vi "Pockels modulation task-Generate data.vi"(8 "error in (no error)":errorcluster, 11 "Setup/Logging queue element":T1={"Imaging Protocol"=enum."Live Imaging", "Number of Trials"=0, "Frame Size"=512, "# Averaged frames"=0, "Dwell time (us)"=0.0, "Index of Z-plane"=0, "Timelapse?"=FALSE, "Logging process is active"=FALSE, "Speed logging enabled"=FALSE, "tdms file ref"=refnum, "path"=path "", "Trial Number"=0, "Expected # points acquired"=FALSE, "Manually stopped"=FALSE, "Last trial"=FALSE, "Ch0 data"=[], "Ch1 data"=[], "Ref Data"=[], "Ref Frame Time"=[], "Image Time"=[], "Continuous Time"=[], "Ref X Length"=0, "Ref Y Length"=0, "# Ref Averaged frames"=0, "Ref Dwell time (us)"=0.0, "Points acquired"={"Ch0 last trial"=0, "Ch1 last trial"=0, "All trials"=0}, "HW Timings File"=refnum} {"Ref Dwell time (us)" format="%#.6g"; "Frame Size" items=["100X100"=100, "128X128"=128, "200X200"=200, "256X256"=256, "512X512"=512, "1024x1024"=1024, "2048x2048"=2048]; "Dwell time (us)" format="%#.6g"}) -> (0 "error":errorcluster, 1 "Data length (points)":i32, 2 "Pockels modulation data":dbl[](graph), 4 "Sampling period (us)":dbl format="%#_6f", 6 "Length of sequence (ms)":dbl format="%#_6f")   [LabVIEW 2020]
uses:
  Typedefs/Logging queue element.ctl
  Typedefs/Imaging Protocols enum.ctl
  Typedefs/Frame Size.ctl
  Typedefs/Acquired points count.ctl
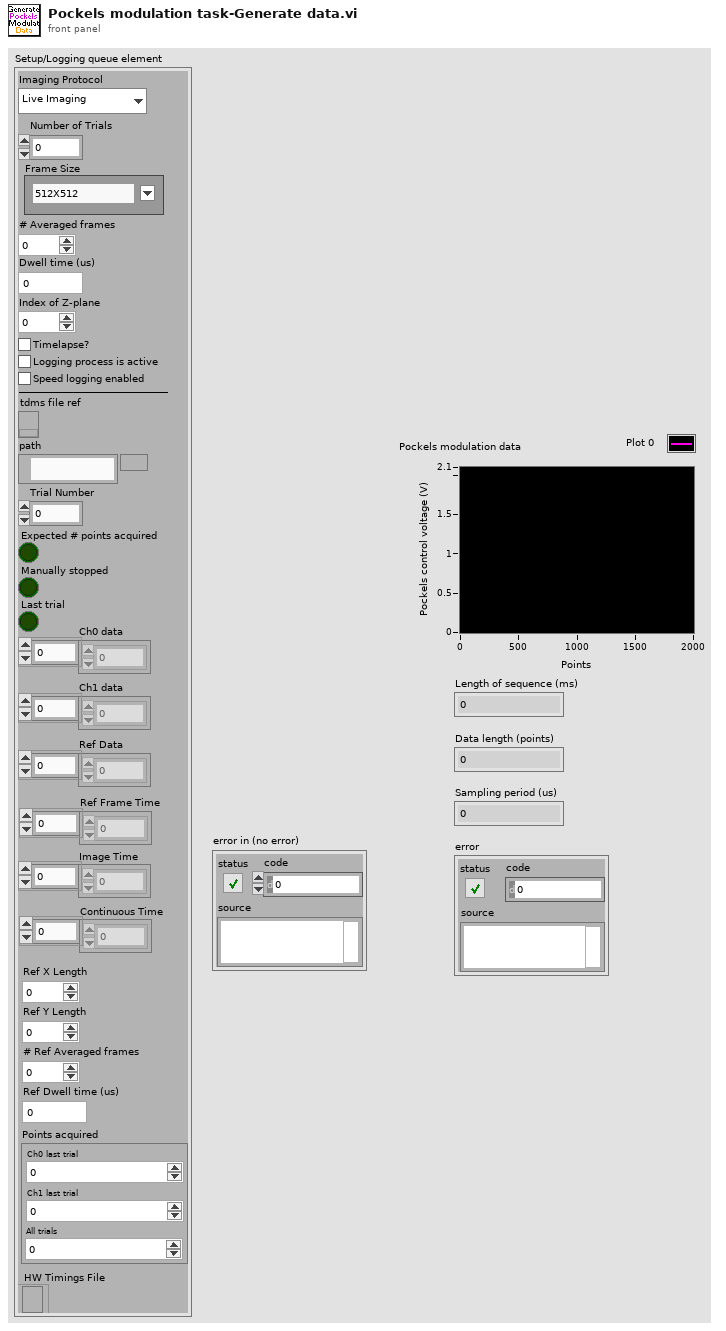
[diagram p1: front panel]
types:
  T1 = typedef "Logging queue element.ctl" = cluster{"Imaging Protocol":T2, "Number of Trials":u16, "Frame Size":T3, "# Averaged frames":u16, "Dwell time (us)":dbl, "Index of Z-plane":i32, "Timelapse?":bool, "Logging process is active":bool, "Speed logging enabled":bool, "tdms file ref":refnum<k34>, "path":path, "Trial Number":i32, "Expected # points acquired":bool, "Manually stopped":bool, "Last trial":bool, "Ch0 data":u32[], "Ch1 data":u32[], "Ref Data":u32[], "Ref Frame Time":u64[], "Image Time":u64[], "Continuous Time":u64[], "Ref X Length":u16, "Ref Y Length":u16, "# Ref Averaged frames":u16, "Ref Dwell time (us)":dbl, "Points acquired":T4, "HW Timings File":refnum<file>}
  T2 = typedef "Imaging Protocols enum.ctl" = enum16{"AOL Z-Stack", "Motor Z Stack", "Functional Acquisition", "Single Plane Acquisition", "Volume Acquisition", "Live Imaging", "Live Plane Imaging", "Live Volume Imaging"}
  T3 = typedef "Frame Size.ctl" = u16
  T4 = typedef "Acquired points count.ctl" = cluster{"Ch0 last trial":u64, "Ch1 last trial":u64, "All trials":u64}
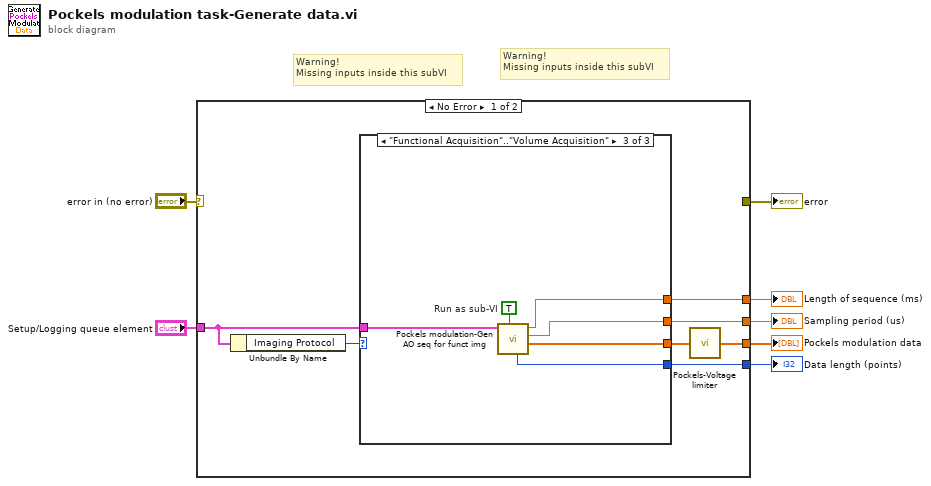
[diagram p0: block diagram]
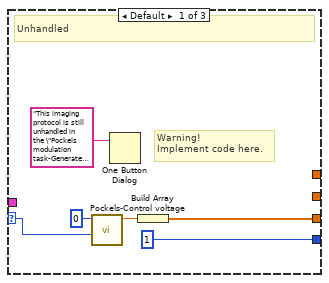
[diagram p2: hidden frame]
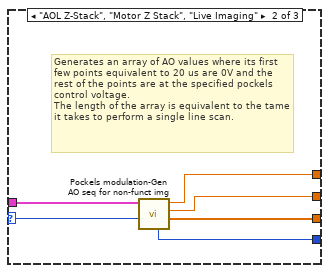
[diagram p3: hidden frame]
diagram:
  # "Warning!\nMissing inputs inside this subVI"
  # "Warning!\nMissing inputs inside this subVI"
  n1 = case shown="No Error" "error in (no error)" {
    selector: "error in (no error)" -> [_ w33]
    tunnel: [w12 _] -> w1
    tunnel: [_ w33] -> w7
    tunnel: [w10 _] -> w5
    tunnel: [w14 _] -> w4
    tunnel: [w13 _] -> w3
    tunnel: "Setup/Logging queue element" -> [w8 _]
    frame No Error {
      n2 = Unbundle By Name(w8) -> ("Imaging Protocol"=w9:T2)
      n3 = case shown="\"Functional Acquisition\"..\"Volume Acquisition\"" w9 {
        selector: w9 -> [w16 w26 _]
        tunnel: [_ w24 w31] -> w14
        tunnel: [_ w23 w30] -> w13
        tunnel: [w19 w22 w28] -> w11
        tunnel: [1 ("upper limit") w21 w27] -> w10
        tunnel: w8 -> [_ w25 w32]
        frame Default {
          # "Warning!\nImplement code here."
          # "Unhandled"
          n4 = call "Pockels-Control voltage.vi"("Imaging Protocol"=w16, "Index of Z-plane"=0) -> ("Pockels control voltage (V)"=w18:dbl)  [unwired: 8 in, 1 out]
          n5 = One Button Dialog(message="This imaging protocol is still unhandled in the \"Pockels modulation task-Generate data.vi\"") -> ()  [unwired: 1 in, 1 out]
          n6 = Build Array(w18) -> (w19:dbl[])
        }
        frame "AOL Z-Stack", "Motor Z Stack", "Live Imaging" {
          # "Generates an array of AO values where its first few points equivalent to 20 us are 0V and the rest of the points are at the specified pockels control voltage.\nThe length of the array is equivalent to the tame it takes to perform a single line scan."
          n7 = call "Pockels modulation-Gen AO seq for non-funct img.vi"("Imaging Protocol"=w26, "Setup/Logging queue element"=w25) -> ("Pockels modulation AO sequence"=w22:dbl[], "Sampling period (us)"=w23:dbl, "Length of sequence (ms)"=w24:dbl, "Data length (points)"=w21:i32)  [unwired: 6 in]
        }
        frame "Functional Acquisition".."Volume Acquisition" {
          w29 = TRUE  # Run as sub-VI
          n8 = call "Pockels modulation-Gen AO seq for funct img.vi"("Run as sub-VI"=w29, "Setup/Logging queue element"=w32) -> ("Pockels modulation sequence"=w28:dbl[], "Sampling period (us)"=w30:dbl, "Sequence length (ms)"=w31:dbl, "Sequence length (points)"=w27:i32)  [unwired: 6 in]
        }
      }
      n9 = call "Pockels-Voltage limiter.vi"("Pockels AO data in"=w11) -> ("Pockels AO data out"=w12:dbl[])
    }
    frame Error {
    }
  }
  "error" <- w7
  "Data length (points)" <- w5
  "Length of sequence (ms)" <- w4
  "Sampling period (us)" <- w3
  "Pockels modulation data" <- w1
